vi "RT Serial Communication Loop.vi"(4 "FPGA version":string="N/A", 5 "RT Main version":string="N/A", 7 "port name in":refnum<visa-resource-name>, 8 "error in":errorcluster, 9 "response queue":refnum<queue>, 10 "message queue":refnum<queue>, 11 "FPGA VI Reference in":refnum<k20>) -> (2 "REQUEST_ID":u64)   [LabVIEW 2018]
uses:
  Message Queue/Message Cluster.ctl
  Type Def Ctrls/RT ctrls/data summary.ctl
  Globals/RT AND FPGA SETTINGS.vi
  Message Queue/Message Queue.lvlib
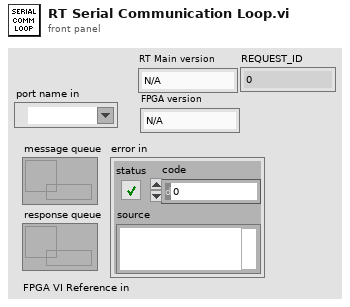
[diagram p1: front panel]
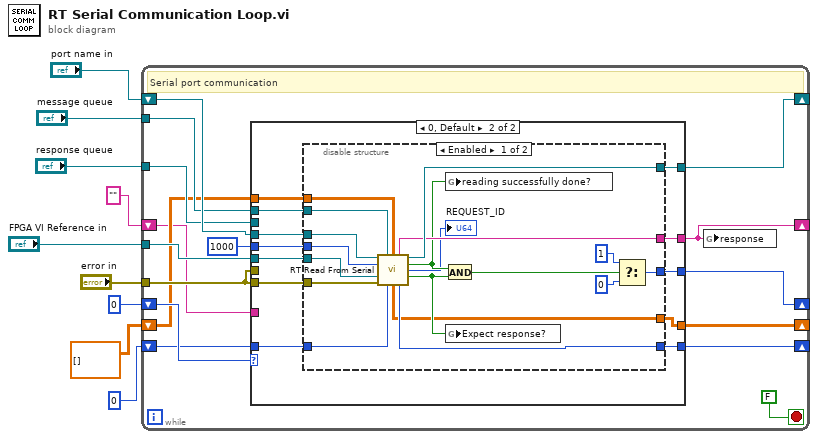
[diagram p0: block diagram]
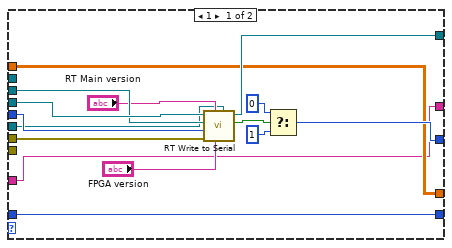
[diagram p2: hidden frame]
diagram:
  n1 = while {
    tunnel: "error in" -> [w20]
    tunnel: "message queue" -> [w23]
    tunnel: "response queue" -> [w18]
    tunnel: "FPGA VI Reference in" -> [w24]
    shift-right: [w17] -> _
    shift-left: "port name in" -> [w25]
    shift-right: [w16] -> _
    shift-left: 0 ("milliseconds to wait") -> [w22]
    shift-right: [w13] -> _
    shift-left: dbl[][] [] -> [w15]
    shift-right: [w12] -> _
    shift-left: 0 -> [w14]
    shift-right: [w10] -> _
    shift-left: "" ("request received") -> [w11]
    stop <- FALSE stop-if-true
    # "Serial port communication"
    n2 = case shown="0, Default" w22 {
      tunnel: w25 -> [w39 w52]
      tunnel: w24 -> [w29 w51]
      tunnel: w20 -> [_ w48]
      tunnel: w23 -> [_ w50]
      tunnel: 1000 ("milliseconds to wait") -> [w35 w49]
      tunnel: w20 -> [w40 _]
      tunnel: w18 -> [w38 _]
      tunnel: [w37 w47] -> w17
      tunnel: [w36 w46] -> w16
      tunnel: w15 -> [w28 w45]
      tunnel: w14 -> [w27 w44]
      tunnel: [w28 w43] -> w13
      tunnel: [w27 w42] -> w12
      tunnel: [w26 w41] -> w10
      tunnel: w11 -> [w26 _]
      frame 1 {
        n3 = call "RT Write to Serial.vi"("FPGA VI Reference in"=w29, "FPGA version"="FPGA version", "RT Main version"="RT Main version", "error in"=w40, "timeout in ms"=w35, "queue in"=w38, "port name in"=w39) -> ("message dequeued?"=w34:bool, "port name out"=w37:refnum<visa-resource-name>)  [unwired: 1 in, 1 out]
        n4 = Select(t=0, s=w34, f=1) -> (s? t:f=w36:i32)
      }
      frame 0, Default {
        n5 = disable-structure shown="Enabled" {
          disable-tunnel: w52 -> [w70 w72]
          disable-tunnel: w51 -> [w69 _]
          disable-tunnel: w50 -> [w68 _]
          disable-tunnel: [w67 w72] -> w47
          disable-tunnel: w49 -> [w66 w71]
          disable-tunnel: [w64 w71] -> w46
          disable-tunnel: w48 -> [w61 _]
          disable-tunnel: w45 -> [w60 _]
          disable-tunnel: w44 -> [w59 _]
          disable-tunnel: [w54 _] -> w43
          disable-tunnel: [w58 _] -> w42
          disable-tunnel: [w57 _] -> w41
          frame Enabled {
            n6 = call "RT Read From Serial.vi"("port name in"=w70, "Message Queue"=w68, "fast output data in"=w60, "timeout (ms)"=w66, "FPGA VI Reference"=w69, "error in (no error)"=w61, "fast output index in"=w59) -> ("request received"=w57:string, "port name out"=w67:refnum<visa-resource-name>, "reading successfully done?"=w56:bool, "REQUEST_ID"=→"REQUEST_ID":u64, "expect response?"=w55:bool, "fast output data out"=w54:dbl[][], "fast output index out"=w58:i32)  [unwired: 1 in, 1 out]
            n7 = And(x=w56, y=w55) -> (x .and. y?=w62:bool)
            n8 = global write "RT AND FPGA SETTINGS.vi" "reading successfully done?"(w56) -> ()
            n9 = global write "RT AND FPGA SETTINGS.vi" "Expect response?"(w55) -> ()
            n10 = Select(t=1, s=w62, f=0) -> (s? t:f=w64:i32)
          }
          frame Disabled {
          }
        }
      }
    }
    n11 = global write "RT AND FPGA SETTINGS.vi" "response"(w10) -> ()
  }
